vi "Query Mulitchannel Configuration.vi"(8 "error in (no error)":errorcluster, 11 "VISA resource name":refnum<visa-resource-name>) -> (0 "error out":errorcluster, 1 "Units in Mulitchannel Operation":i32, 2 "Enabled Channels":string="\"\"", 3 "VISA resource name out":refnum<visa-resource-name>)   [LabVIEW 2023]
doc: "Returns the number of units in master-slave parallel operation and the valid channels as a comma-separated list."
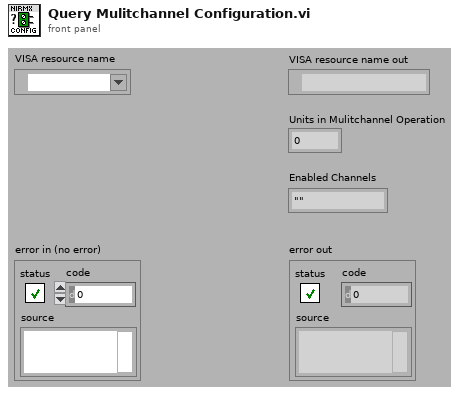
[diagram p1: front panel]
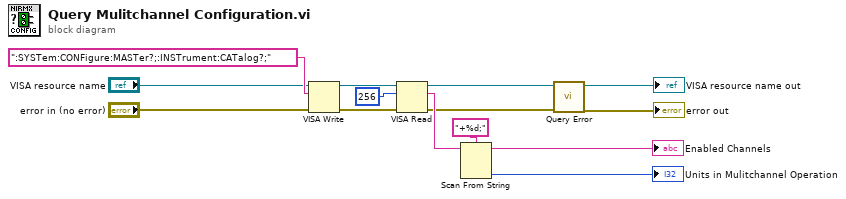
[diagram p0: block diagram]
diagram:
  n1 = VISA Write(VISA resource name="VISA resource name", write buffer=":SYSTem:CONFigure:MASTer?;:INSTrument:CATalog?;", error in (no error)="error in (no error)") -> (VISA resource name out=w8:refnum<visa-resource-name>, error out=w9:errorcluster)  [unwired: 1 out]
  n2 = VISA Read(VISA resource name=w8, byte count=u32 256, error in (no error)=w9) -> (VISA resource name out=w2:refnum<visa-resource-name>, read buffer=w6:string, error out=w1:errorcluster)  [unwired: 1 out]
  n3 = Scan From String(format string="+%d;", input string=w6) -> (remaining string=→"Enabled Channels":string, output 1=→"Units in Mulitchannel Operation":i32)  [unwired: 3 in, 2 out]
  n4 = call "Query Error.vi"("error in (no error)"=w1, "VISA resource name"=w2) -> ("error out"=→"error out":errorcluster, "VISA resource name out"=→"VISA resource name out":refnum<visa-resource-name>)  [unwired: 6 in, 2 out]
